vi "CreateRefs.vi"(8 "error in (no error)":errorcluster) -> (0 "error out":errorcluster, 3 "Cluster":T1)   [LabVIEW 2019, in "lv-providershell-example2.lvlib"]
uses:
  lv-providershell-example2.lvlib
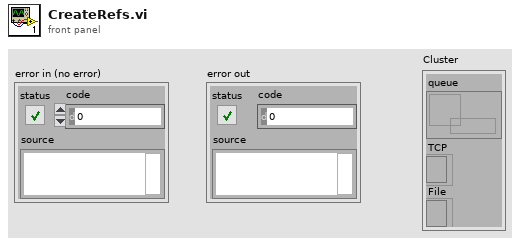
[diagram p1: front panel]
types:
  T1 = cluster{"queue":refnum<queue>, "TCP":refnum<k5>, "File":refnum<file>}
  T2 = enum16{"open", "replace", "create", "open or create", "replace or create", "replace or create with confirmation"}
  T3 = cluster{"queue out":refnum<queue>, "connection ID":refnum<k5>, "refnum out":refnum<file>}
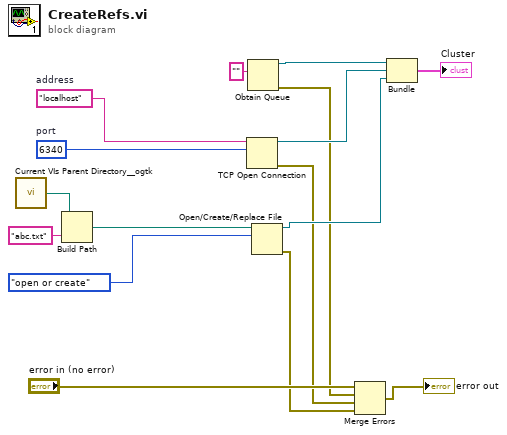
[diagram p0: block diagram]
diagram:
  w6 = u16 6340  # port
  w7 = "localhost"  # address
  n1 = call <userlib>:"Current VIs Parent Directory__ogtk.vi"() -> ("Parent Directory (+ Relative)"=w14:path)  [unwired: 5 in]
  n2 = Build Path(base path=w14, name or relative path="abc.txt") -> (appended path=w12:path)
  n3 = TCP Open Connection(address=w7, remote port or service name=w6) -> (connection ID=w5:refnum<k5>, error out=w2:errorcluster)  [unwired: 3 in]
  n4 = Obtain Queue(element data type="" ("name (unnamed)")) -> (queue out=w10:refnum<queue>, error out=w3:errorcluster)  [unwired: 4 in, 1 out]
  n5 = Open/Create/Replace File(file path (use dialog)=w12, operation (0:open)=T2."open or create") -> (refnum out=w9:refnum<file>, error out=w1:errorcluster)  [unwired: 4 in, 1 out]
  n6 = Merge Errors("error in (no error)", w3, w2, w1) -> (→"error out":errorcluster)
  n7 = Bundle("queue out"=w10, "connection ID"=w5, "refnum out"=w9) -> (→"Cluster":T3)  [unwired: 1 in]
